vi "Image To Array.vi"() -> ()   [LabVIEW 2014]
doc: "This example shows how to convert an image into a two-dimensional LabVIEW array. By converting an image into a LabVIEW array, you can apply all the analysis, display, and array operators available in LabVIEW to the image data."
panel:
  in  "Optional Rectangle":i32[](array[numeric])=[98, 180, 115, 197]
  out "Image Source":T1(plugin-control)
  out "Pixels Values":u8[][](array[numeric])
  # "Overview: Demonstrates how to retrieve an array of pixel values from an image.\nRequirements: NI Vision Development Module\nInstructions: Run the VI."
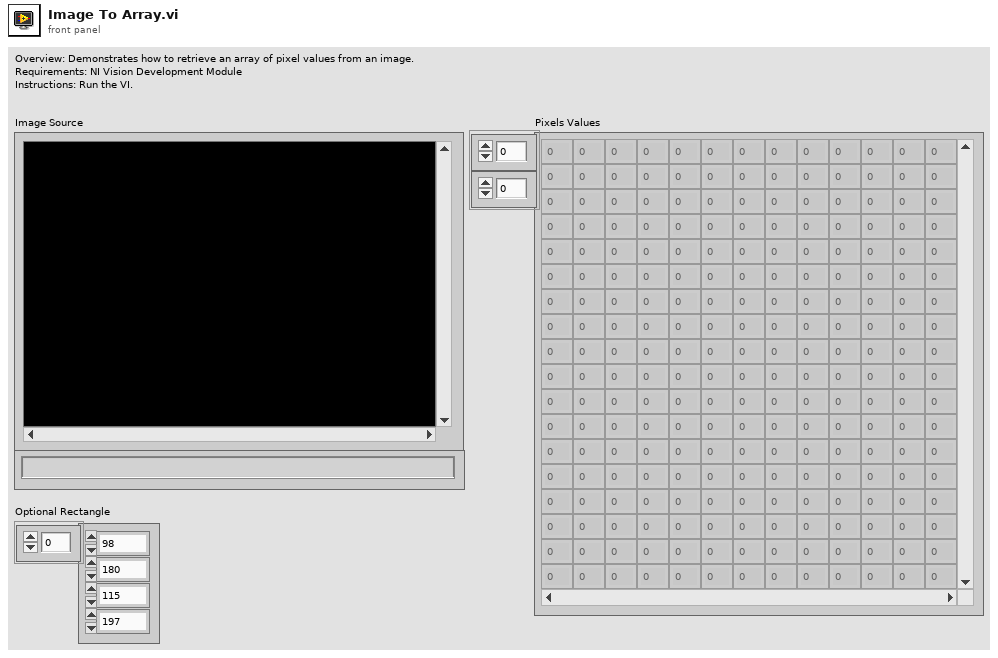
[diagram p1: front panel]
types:
  T1 = typedef "IMAQ Image.ctl" = refnum<image>
  T2 = typedef "Image Type" = u32
  T3 = cluster{"Optional Rectangle[0]":i32, "Optional Rectangle[1]":i32, "Optional Rectangle[2]":i32, "Optional Rectangle[3]":i32, "Optional Rectangle[4]":i32}
  T4 = typedef "ROI Descriptor" = cluster{"Global Rectangle":i32[], "Contours":cluster{"ID":enum32{"External", "Internal"}, "Type":u32, "Coordinates":i32[]}[]}
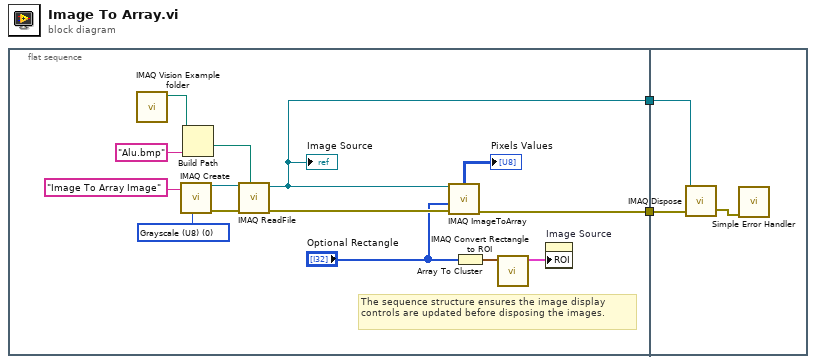
[diagram p0: block diagram]
diagram:
  n1 = flat-sequence {
    tunnel: [w7] -> w2
    tunnel: [w6] -> w1
    tunnel: w2 -> [w18]
    tunnel: w1 -> [w17]
    frame #0 {
      w9 = T2 0 items=["Grayscale (U8)", "Grayscale (I16)", "Grayscale (SGL)", "Complex (CSG)", "RGB (U32)", "HSL (U32)", "RGB (U64)", "Grayscale (U16)"] ("Image Type")
      # "The sequence structure ensures the image display controls are updated before disposing the images."
      n2 = call "IMAQ Vision Example folder.vi"() -> ("Example Image Path"=w14:path)  [unwired: 11 in]
      n3 = call "IMAQ Create"("Image Name"="Image To Array Image", "Image Type"=w9) -> ("New Image"=w12:T1, "error out"=w13:errorcluster)  [unwired: 3 in]
      n4 = Build Path(base path=w14, name or relative path="Alu.bmp") -> (appended path=w11:path)
      n5 = call "IMAQ ReadFile"("File Path"=w11, "error in (no error)"=w13, "Image"=w12) -> ("error out"=w8:errorcluster, "Image Out"=w6:T1)  [unwired: 4 in, 3 out]
      "Image Source" <- w6
      n6 = call "IMAQ ImageToArray"("error in (no error)"=w8, "Optional Rectangle"="Optional Rectangle", "Image"=w6) -> ("error out"=w7:errorcluster, "Image Pixels (U8)"=→"Pixels Values":u8[][])  [unwired: 1 in, 3 out]
      n7 = Array To Cluster(array="Optional Rectangle") -> (cluster=w4:T3)
      n8 = call "IMAQ Convert Rectangle to ROI"("Rectangle"=w4) -> ("ROI Descriptor"=w3:T4)  [unwired: 8 in, 1 out]
      n9 = property on="Image Source" class="ImageControl"("ROI"=w3) -> ()  [unwired: 2 in, 2 out]
    }
    frame #1 {
      n10 = call "IMAQ Dispose"("Image"=w17, "error in (no error)"=w18) -> ("error out"=w19:errorcluster)  [unwired: 4 in]
      n11 = call <vilib>:"Simple Error Handler.vi"("error in (no error)"=w19) -> ()  [unwired: 4 in, 5 out]
    }
  }
